vi "LED Configure.vi"(9 "LED On":bool, 10 "refnum name":string, 11 "LEDChannel":T1) -> ()   [LabVIEW 2019]
uses:
  <vilib>/Rock Robotics/WPI/ThirdParty/Phoenix-LabVIEW/CANifier/CTRE_CANifier_LEDChannel.ctl
  mOS_XIII/MoS_XIII/Globals/LED_Globals.vi
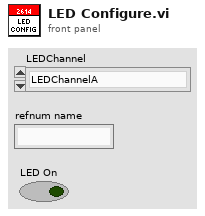
[diagram p1: front panel]
types:
  T1 = typedef "CTRE_CANifier_LEDChannel.ctl" = enum32{"LEDChannelA", "LEDChannelB", "LEDChannelC"}
  T2 = typedef "CTRE_CANifier_DeviceRef.ctl" = cluster{"DeviceStatus":errorcluster, "Device Number":u8, "Handle":u64, "UsageFrame":u32, "Library Path":path}
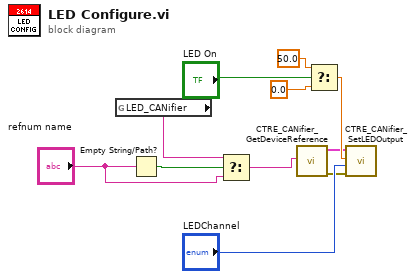
[diagram p0: block diagram]
diagram:
  n1 = global read "LED_Globals.vi" "LED_CANifier"() -> (w3:string)
  n2 = Empty String/Path?(string/path="refnum name") -> (empty?=w4:bool)
  n3 = Select(t=w3, s=w4, f="refnum name") -> (s? t:f=w1:string)
  n4 = call <vilib>:"CTRE_CANifier_GetDeviceReference.vi"("refnum name"=w1) -> ("error out"=w6:errorcluster, "CANifierDevRef"=w5:T2)  [unwired: 9 in]
  n5 = Select(t=50.0, s="LED On", f=0.0) -> (s? t:f=w11:dbl)
  n6 = call <vilib>:"CTRE_CANifier_SetLEDOutput.vi"("error in"=w6, "LEDChannel"="LEDChannel", "Percent Output"=w11, "CANifierDevRef"=w5) -> ()  [unwired: 6 in, 2 out]
